vi "UI.vi"(8 "error in (no error)":errorcluster, 11 "Subtract in":refnum<class "Subtract.lvclass">) -> (0 "error out":errorcluster, 3 "Subtract out":refnum<class "Subtract.lvclass">)   [LabVIEW 2020, in "Subtract.lvclass"]
uses:
  Subtract.lvclass
  C:/Users/Khishore/Downloads/Assignment 25 3/Assignment 25/Arithmetic Operations/Arithmetic Operations.lvclass
  Typedefs/User event operations.ctl
  Arithmetic Operations.lvclass/Arithmetic Operations.ctl
  Accessors/Write/Write A.vi
  Accessors/Write/Write B.vi
  Accessors/Read/Read C.vi
  Accessors/Read/Read A.vi
  Accessors/Read/Read B.vi
  Simple calculator.lvlib
panel:
  out "C":dbl
  in  "B":dbl
  in  "A":dbl
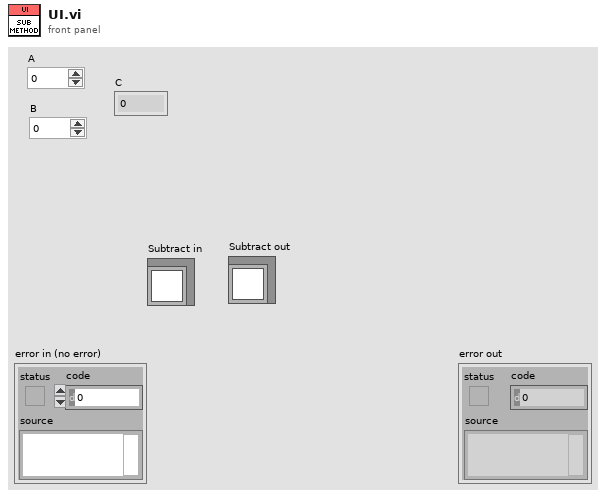
[diagram p1: front panel]
types:
  T1 = typedef "Simple calculator.lvlib/User event operations.ctl" = enum16{"Create", "Get Ref", "Generate ", "Destroy"}
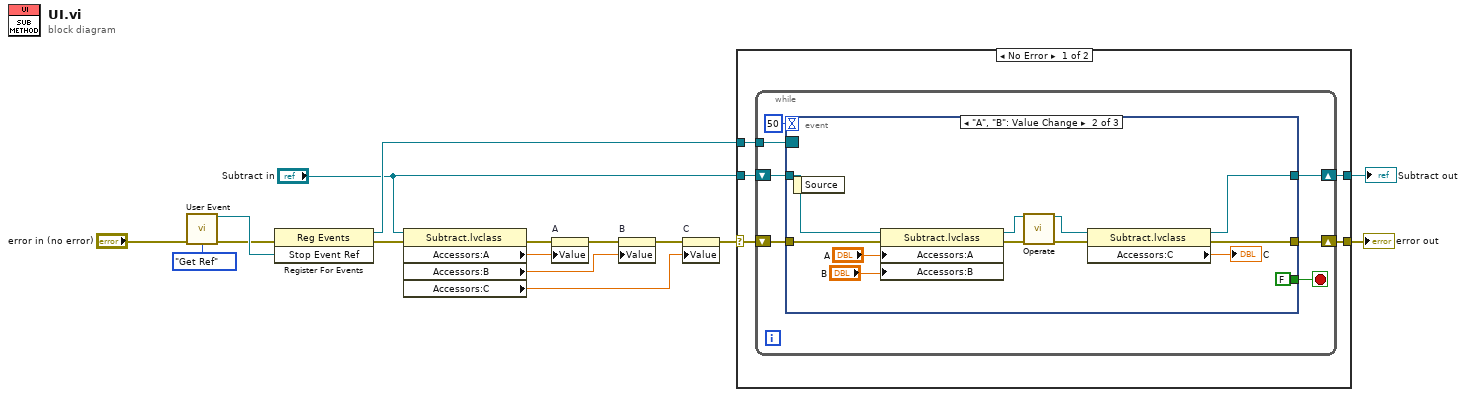
[diagram p0: block diagram]
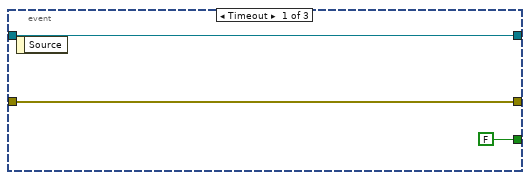
[diagram p2: hidden frame]
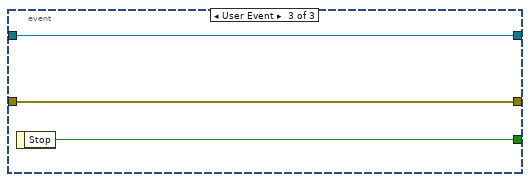
[diagram p3: hidden frame]
diagram:
  n1 = call "User Event.vi"("Error in"="error in (no error)", "Operation"=User_event_operations."Get Ref") -> ("Stop Event Ref"=w15:refnum<user-event>, "Error out"=w14:errorcluster)  [unwired: 12 in]
  n2 = register-events(error in=w14, w15) -> (reference out=w12:refnum<event-registration>, error out=w11:errorcluster)  [unwired: 1 in]
  n3 = property class="Subtract.lvclass"(reference="Subtract in", error in=w11) -> (error out=w9:errorcluster, "Accessors:A"=w5:dbl, "Accessors:B"=w4:dbl, "Accessors:C"=w3:dbl)  [unwired: 1 out]
  n4 = property on="A" class="DigNum (strict)"(error in=w9, "Value"=w5) -> (error out=w8:errorcluster)  [unwired: 1 in, 1 out]
  n5 = property on="B" class="DigNum (strict)"(error in=w8, "Value"=w4) -> (error out=w7:errorcluster)  [unwired: 1 in, 1 out]
  n6 = property on="C" class="DigNum (strict)"(error in=w7, "Value"=w3) -> (error out=w6:errorcluster)  [unwired: 1 in, 1 out]
  n7 = case shown="No Error" w6 {
    selector: w6 -> [w21 w47]
    tunnel: [w17 w48] -> w16
    tunnel: "Subtract in" -> [w18 w48]
    tunnel: w12 -> [w20 _]
    tunnel: [w19 w47] -> w2
    frame No Error {
      n8 = while {
        tunnel: w20 -> [w26]
        shift-right: [w23] -> w17
        shift-left: w18 -> [w24]
        shift-right: [w25] -> w19
        shift-left: w21 -> [w27]
        stop <- w22 stop-if-true
        n9 = event shown="[1] \"A\", \"B\": Value Change" {
          selector: w26 -> [_ _ _]
          dyn-events: _ -> [_ _ _]
          timeout: 50 -> [_ _ _]
          tunnel: w27 -> [w31 w43 w45]
          tunnel: [w31 w34 w45] -> w25
          tunnel: [w30 w33 w44] -> w23
          tunnel: w24 -> [w30 w42 w44]
          tunnel: [FALSE ("Stop") FALSE ("Stop") w46] -> w22
          event Timeout {
            n10 = event-data() -> ()  [unwired: 1 in, 1 out]
          }
          event "A", "B": Value Change {
            n11 = event-data() -> ()  [unwired: 1 in, 1 out]
            n12 = property class="Subtract.lvclass"(reference=w42, error in=w43, "Accessors:A"="A", "Accessors:B"="B") -> (reference out=w38:refnum<class "Subtract.lvclass">, error out=w39:errorcluster)
            n13 = call-dynamic "Operate.vi"("Subtract in"=w38, "error in (no error)"=w39) -> ("Subtract out"=w37:refnum<class "Subtract.lvclass">, "error out"=w36:errorcluster)  [unwired: 12 in]
            n14 = property class="Subtract.lvclass"(reference=w37, error in=w36) -> (reference out=w33:refnum<class "Subtract.lvclass">, error out=w34:errorcluster, "Accessors:C"=→"C":dbl)
          }
          event User Event {
            n15 = event-data() -> ("Stop"=w46:bool)  [unwired: 1 in]
          }
        }
      }
    }
    frame Error {
    }
  }
  "error out" <- w2
  "Subtract out" <- w16
